vi "sampling_theorem.vi"() -> ()   [LabVIEW 2017]
uses:
  <vilib>/express/express shared/transition.llb/Dynamic To Waveform Array.vi
  <vilib>/express/express signal manip/GetorSetDDTAttributes/Set DDT Attributes/SetT0.vi
  <vilib>/express/express shared/transition.llb/Waveform Array To Dynamic.vi
  <vilib>/express/express signal manip/GetorSetDDTAttributes/Set DDT Attributes/Set DDT Properties.xnode
panel:
  in  "Signal type":enum16{"Sine", "Square", "Triangle", "Sawtooth"}(ring)
  in  "signal frequency [Hz]:":dbl=100.0 caption="dt" min=1.0 max=1000.0
  out "Waveform Graph 3":dynamicdata(graph)
  in  "sampling frequency [Hz]:":dbl=1000.0 caption="dt"
  out "Reconstructed":dynamicdata(graph) caption="Resampled Signals"
  out "Decimated":dynamicdata(graph) caption="Resampled Signals"
  out "IN":dynamicdata(graph)
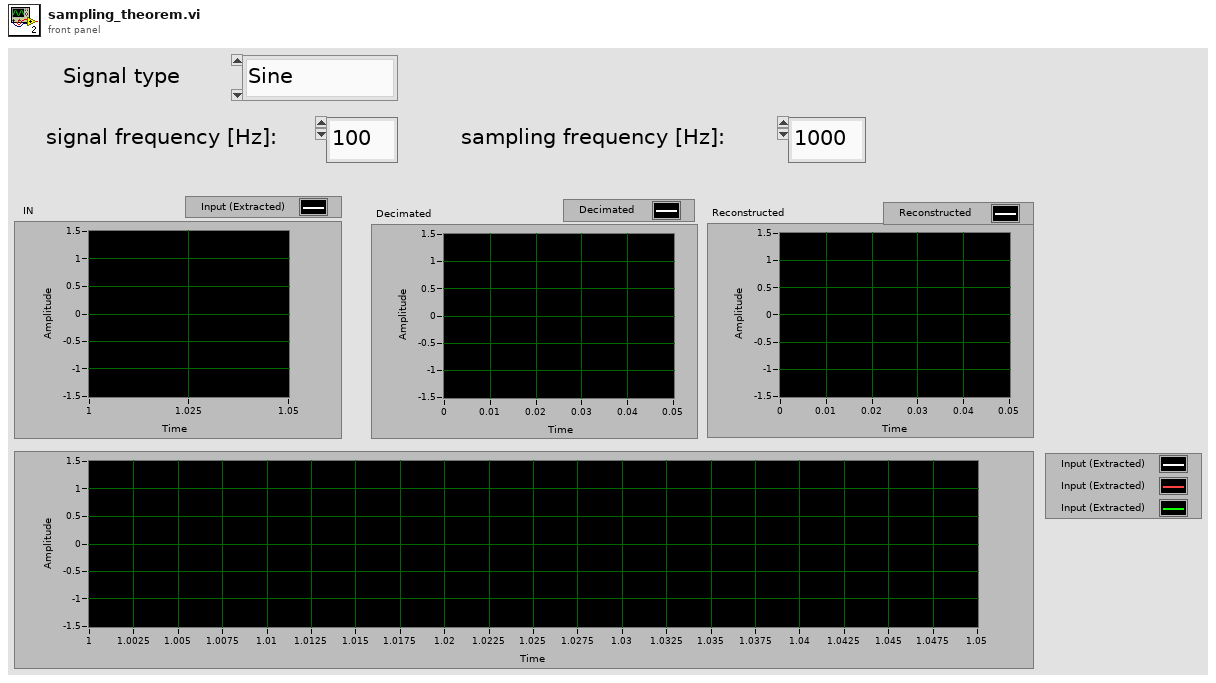
[diagram p1: front panel]
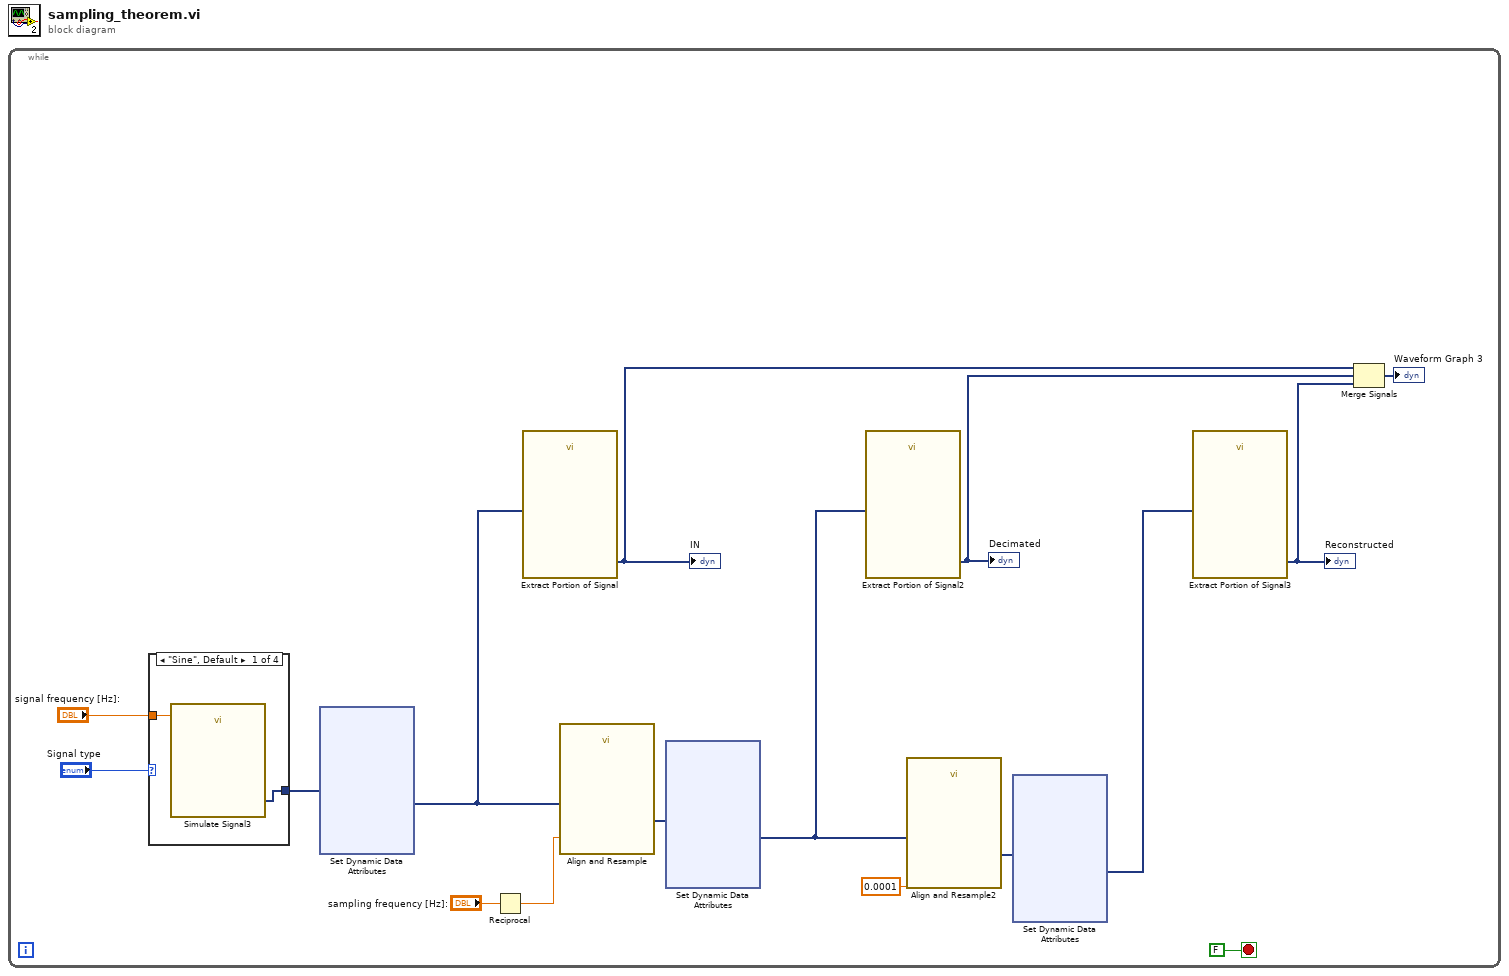
[diagram p0: block diagram]
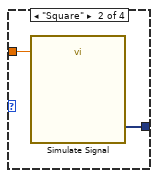
[diagram p2: hidden frame]
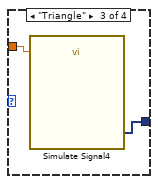
[diagram p3: hidden frame]
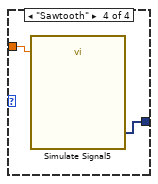
[diagram p4: hidden frame]
diagram:
  n1 = while {
    stop <- FALSE stop-if-true
    n2 = case shown="\"Sine\", Default" "Signal type" {
      tunnel: [w17 w20 w21 w23] -> w14
      tunnel: "signal frequency [Hz]:" -> [w18 w19 w22 w24]
      frame "Sine", Default {
        n3 = call "Simulate Signal3"("Frequency"=w18) -> ("Sine"=w17:dynamicdata)  [unwired: 13 in, 1 out]
      }
      frame "Square" {
        n4 = call "Simulate Signal"("Frequency"=w19) -> ("Square"=w20:dynamicdata)  [unwired: 13 in, 1 out]
      }
      frame "Triangle" {
        n5 = call "Simulate Signal4"("Frequency"=w22) -> ("Triangle"=w21:dynamicdata)  [unwired: 13 in, 1 out]
      }
      frame "Sawtooth" {
        n6 = call "Simulate Signal5"("Frequency"=w24) -> ("Sawtooth"=w23:dynamicdata)  [unwired: 13 in, 1 out]
      }
    }
    n7 = xnode "Set Dynamic Data Attributes"("Signals In"=w14) -> ("Signals Out"=w7:dynamicdata)  [unwired: 3 in, 1 out]
    n8 = Reciprocal(x="sampling frequency [Hz]:") -> (1/x=w11:dbl)
    n9 = call "Extract Portion of Signal"("Signals"=w7) -> ("Section"=w6:dynamicdata)  [unwired: 9 in, 1 out]
    "IN" <- w6
    n10 = call "Align and Resample"("dt"=w11, "Signals"=w7) -> ("Resampled Signals"=w15:dynamicdata)  [unwired: 7 in, 2 out]
    n11 = xnode "Set Dynamic Data Attributes"("Signals In"=w15) -> ("Signals Out"=w10:dynamicdata)  [unwired: 3 in, 1 out]
    n12 = call "Extract Portion of Signal2"("Signals"=w10) -> ("Section"=w5:dynamicdata)  [unwired: 9 in, 1 out]
    "Decimated" <- w5
    n13 = call "Align and Resample2"("dt"=0.0001 ("dt 2"), "Signals"=w10) -> ("Resampled Signals"=w13:dynamicdata)  [unwired: 7 in, 2 out]
    n14 = xnode "Set Dynamic Data Attributes"("Signals In"=w13) -> ("Signals Out"=w9:dynamicdata)  [unwired: 3 in, 1 out]
    n15 = call "Extract Portion of Signal3"("Signals"=w9) -> ("Section"=w4:dynamicdata)  [unwired: 9 in, 1 out]
    "Reconstructed" <- w4
    n16 = Merge Signals(w6, w5, w4) -> (→"Waveform Graph 3":dynamicdata)
  }
